vi "Transform3d_Plus.vi"(9 "otherTransform3d":T1={"TRANSLATION3D"={"X"=0.0, "Y"=0.0, "Z"=0.0}, "ROTATION3D"={"Q_quaternion"={"R"=1.0, "V"=[0.0, 0.0, 0.0]}}, "XF"=FALSE} {"TRANSLATION3D"."Z" format="%14.3f"; "TRANSLATION3D"."Y" format="%14.3f"; "TRANSLATION3D"."X" format="%14.3f"}, 11 "in Transform3d":T1={"TRANSLATION3D"={"X"=0.0, "Y"=0.0, "Z"=0.0}, "ROTATION3D"={"Q_quaternion"={"R"=1.0, "V"=[0.0, 0.0, 0.0]}}, "XF"=FALSE} {"TRANSLATION3D"."Z" format="%14.3f"; "TRANSLATION3D"."Y" format="%14.3f"; "TRANSLATION3D"."X" format="%14.3f"}) -> (3 "Transform3d":T1={"TRANSLATION3D"={"X"=0.0, "Y"=0.0, "Z"=0.0}, "ROTATION3D"={"Q_quaternion"={"R"=1.0, "V"=[0.0, 0.0, 0.0]}}, "XF"=FALSE} {"TRANSLATION3D"."Z" format="%14.3f"; "TRANSLATION3D"."Y" format="%14.3f"; "TRANSLATION3D"."X" format="%14.3f"})   [LabVIEW 2019, in "Trajectory_Library.lvlib"]
doc: "Composes two transformations.\n\nParameters:\n - IN TRANSFORM3d -- This TRANSFORM data structure\n - other Transform3d -- The transform to compose with this one.\n\nResults:\n - OUT TRANSFORM3d -- The composition of the two transformations."
uses:
  Trajectory_Library.lvlib
  TRANSFORM3D.ctl
  TRANSLATION3D.ctl
  ROTATION3D.ctl
  QUATERNION.ctl
  Pose3d_New_Trans3dRot3d.vi
  Translation3d_Create_Default.vi
  Rotation3d_Create_Default.vi
  Transform3d_Create_Trans3dRot3d.vi
  Translation3d_Minus.vi
  Translation3d_RotateBy.vi
  Rotation3d_UnaryMinus.vi
  Pose3d_getTranslation3d.vi
  Pose3d_getRotation3d.vi
  Rotation3d_Minus.vi
  Transform3d_GetTranslation3d.vi
  Transform3d_GetRotation3d.vi
  Translation3d_Plus.vi
  Rotation3d_Plus.vi
  Quaternion_New_Default.vi
  Translation3d_Create.vi
  Rotation3d_GetQuaterion.vi
  Quaternion_New.vi
  Quaternion_Times.vi
  Quaternion_Inverse.vi
  Quaternion_Get_All.vi
  Rotation3d_Create_Quaternion.vi
  Rotation3d_RotateBy.vi
  Quaternion_Normalize.vi
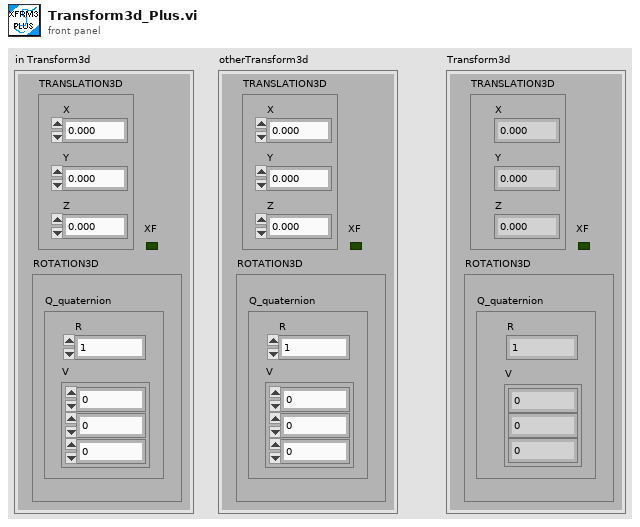
[diagram p1: front panel]
types:
  T1 = typedef "Trajectory_Library.lvlib/TRANSFORM3D.ctl" = cluster{"TRANSLATION3D":T2, "ROTATION3D":T3, "XF":bool}
  T2 = typedef "Trajectory_Library.lvlib/TRANSLATION3D.ctl" = cluster{"X":dbl, "Y":dbl, "Z":dbl}
  T3 = typedef "Trajectory_Library.lvlib/ROTATION3D.ctl" = cluster{"Q_quaternion":T4}
  T4 = typedef "Trajectory_Library.lvlib/QUATERNION.ctl" = cluster{"R":dbl, "V":dbl[]}
  T5 = typedef "Trajectory_Library.lvlib/POSE3D.ctl" = cluster{"Translation3d":T2, "Rotation3d":T3}
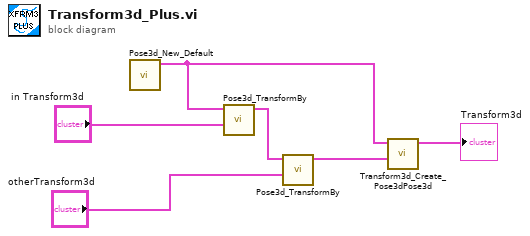
[diagram p0: block diagram]
diagram:
  n1 = call "Pose3d_New_Default.vi"() -> ("outPose3d"=w6:T5)  [unwired: 11 in]
  n2 = call "Pose3d_TransformBy.vi"("other Transform3d"="in Transform3d", "in Pose3d"=w6) -> ("out POSE3d"=w5:T5)  [unwired: 9 in]
  n3 = call "Pose3d_TransformBy.vi"("other Transform3d"="otherTransform3d", "in Pose3d"=w5) -> ("out POSE3d"=w4:T5)  [unwired: 9 in]
  n4 = call "Transform3d_Create_Pose3dPose3d.vi"("last Pose3d"=w4, "initial Pose3d"=w6) -> ("Transform3d"=→"Transform3d":T1)  [unwired: 9 in]
